vi "Read sync data.vi"(8 "error in (no error)":errorcluster, 11 "Shared Memory runtime in":refnum<class "Shared Memory runtime.lvclass">) -> (0 "error out":errorcluster, 2 "sync data":T1, 3 "Shared Memory runtime out":refnum<class "Shared Memory runtime.lvclass">)   [LabVIEW 2013, in "Shared Memory runtime.lvclass"]
uses:
  Shared Memory runtime.lvclass
  controls/sync data.ctl
  controls/semaphore data.ctl
  <vilib>/NI/NI Linux RT IPC/POSIX Threads/Classes/Semaphore/Controls/reference.ctl
  <vilib>/NI/NI Linux RT IPC/POSIX Threads/Classes/Semaphore/Semaphore.lvclass
  <vilib>/NI/NI Linux RT IPC/Shared Memory/Classes/Shared Memory/Public/Controls/reference.ctl
  <vilib>/NI/NI Linux RT IPC/Shared Memory/Classes/Shared Memory/Shared Memory.lvclass
  controls/sync timing indices.ctl
  controls/sync timing pointers.ctl
  Shared Memory runtime.lvclass/Shared Memory runtime.ctl
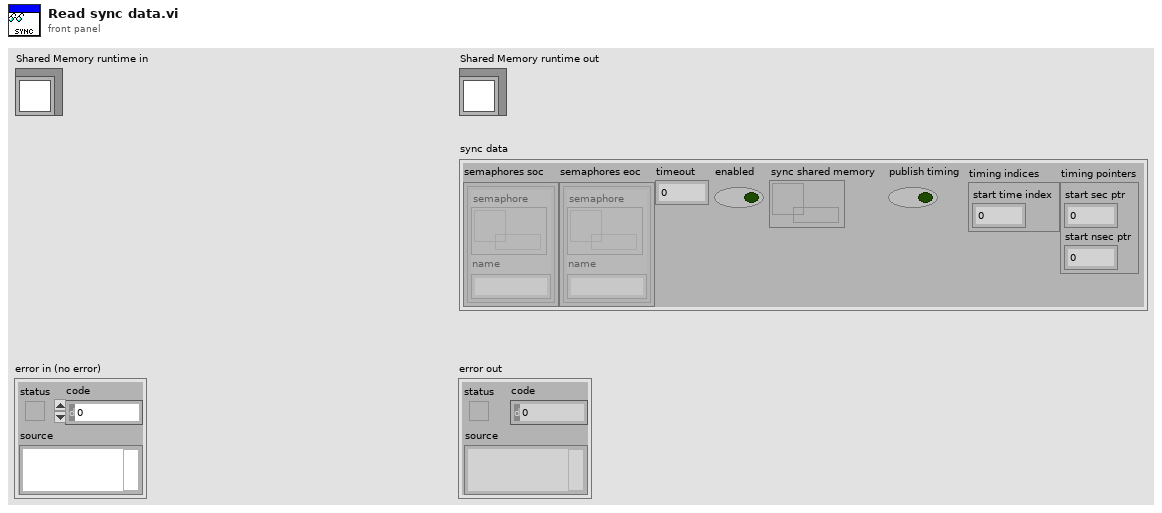
[diagram p1: front panel]
types:
  T1 = typedef "Shared Memory runtime.lvclass/sync data.ctl" = cluster{"semaphores soc":T2[], "semaphores eoc":T2[], "timeout":dbl, "enabled":bool, "sync shared memory":T4, "publish timing":bool, "timing indices":T5, "timing pointers":T6}
  T2 = typedef "Shared Memory runtime.lvclass/semaphore data.ctl" = cluster{"semaphore":T3, "name":string}
  T3 = typedef "POSIX Threads.lvlib/Semaphore.lvclass/reference.ctl" = refnum<data-value>
  T4 = typedef "Shared Memory.lvlib/Shared Memory.lvclass/reference.ctl" = refnum<data-value>
  T5 = typedef "Shared Memory runtime.lvclass/sync timing indices.ctl" = cluster{"start time index":i32}
  T6 = typedef "Shared Memory runtime.lvclass/sync timing pointers.ctl" = cluster{"start sec ptr":u64, "start nsec ptr":u64}
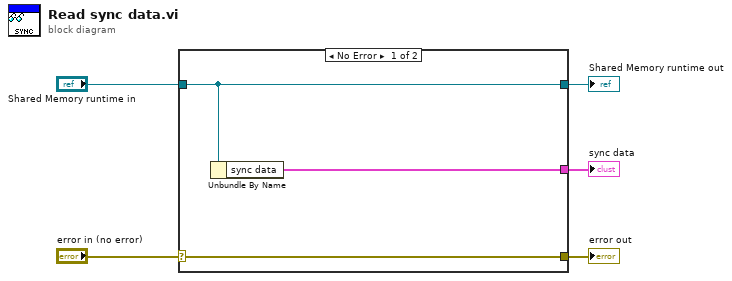
[diagram p0: block diagram]
diagram:
  n1 = case shown="No Error" "error in (no error)" {
    selector: "error in (no error)" -> [w8 w9]
    tunnel: [w8 w9] -> w4
    tunnel: [w7 w10] -> w2
    tunnel: "Shared Memory runtime in" -> [w7 w10]
    tunnel: [w6 _] -> w1
    frame No Error {
      n2 = Unbundle By Name(w7) -> ("sync data"=w6:T1)
    }
    frame Error {
    }
  }
  "error out" <- w4
  "Shared Memory runtime out" <- w2
  "sync data" <- w1
